vi "Create TopicFilter.vi"(5 "TopicFilter in":refnum<class "TopicFilter.lvclass">, 8 "error in (no error)":errorcluster, 11 "Topic Filter":string) -> (0 "error out":errorcluster, 3 "TopicFilter out":refnum<class "TopicFilter.lvclass">)   [LabVIEW 2013, in "MQTT Server.lvlib" / "TopicFilter.lvclass"]
uses:
  TopicFilter.lvclass
  TopicFilter.lvclass/TopicFilter.ctl
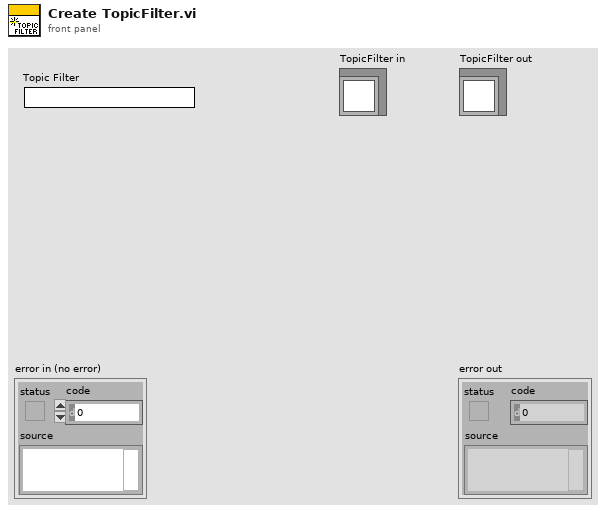
[diagram p1: front panel]
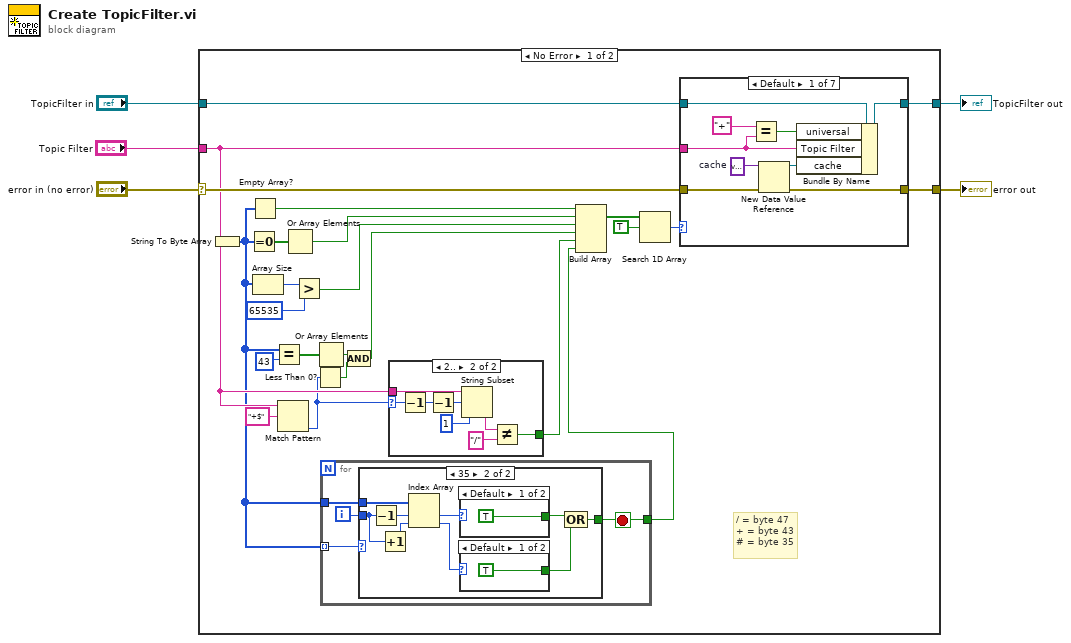
[diagram p0: block diagram]
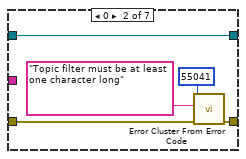
[diagram p6: hidden frame]
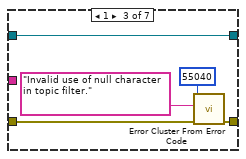
[diagram p7: hidden frame]
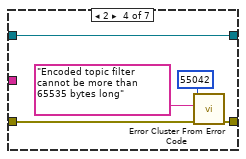
[diagram p8: hidden frame]
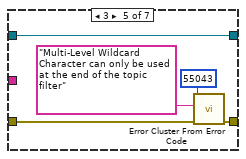
[diagram p9: hidden frame]
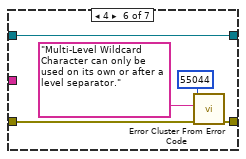
[diagram p10: hidden frame]
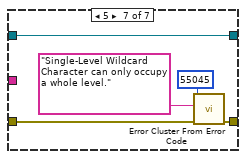
[diagram p11: hidden frame]
diagram:
  n1 = case shown="No Error" "error in (no error)" {
    selector: "error in (no error)" -> [w27 w93]
    tunnel: [w26 w93] -> w4
    tunnel: [w28 w92] -> w2
    tunnel: "TopicFilter in" -> [w29 w92]
    tunnel: "Topic Filter" -> [w10 _]
    frame No Error {
      # "/ = byte 47\n+ = byte 43\n# = byte 35"
      n2 = String To Byte Array(string=w10) -> (unsigned byte array=w7:u8[])
      n3 = Equal To 0?(x=w7) -> (x = 0?=w25:bool[])
      n4 = Empty Array?(array=w7) -> (empty?=w24:bool)
      n5 = Array Size(array=w7) -> (size(s)=w19:i32)
      n6 = Equal?(x=w7, y=u8 43) -> (x = y?=w14:bool[])
      n7 = Match Pattern(string=w10, regular expression="+$") -> (offset past match=w9:i32)  [unwired: 1 in, 3 out]
      n8 = Or Array Elements(Boolean array=w25) -> (logical OR=w23:bool)
      n9 = Greater?(x=w19, y=65535) -> (0:w17:bool)
      n10 = Less Than 0?(x=w9) -> (x < 0?=w12:bool)
      n11 = Or Array Elements(Boolean array=w14) -> (logical OR=w13:bool)
      n12 = for {
        tunnel: w7 -> [w33] mode=indexing
        tunnel: w7 -> [w32]
        tunnel: [w30] -> w6
        i -> [w31]
        stop <- w30 stop-if-true
        n13 = case shown="35" w33 {
          tunnel: w32 -> [_ w42]
          tunnel: w31 -> [_ w40]
          tunnel: [_ w34] -> w30
          frame Default {
          }
          frame 35 {
            n14 = Decrement(x=w40) -> (x-1=w41:i32)
            n15 = Increment(x=w40) -> (x+1=w39:i32)
            n16 = Index Array(array=w42, index #1=w41, index #2=w39) -> (element #1=w38:u8, element #2=w37:u8)
            n17 = case shown="Default" w38 {
              tunnel: [TRUE _] -> w36
              frame Default {
              }
              frame 0, 47 {
              }
            }
            n18 = case shown="Default" w37 {
              tunnel: [TRUE _] -> w35
              frame Default {
              }
              frame 0, 47 {
              }
            }
            n19 = Compound Arithmetic op=OR(w36, w35) -> (w34:bool)
          }
        }
      }
      n20 = Compound Arithmetic op=AND(w13, w12) -> (w11:bool)
      n21 = case shown="2.." w9 {
        selector: w9 -> [_ w48]
        tunnel: w10 -> [_ w52]
        tunnel: [_ w45] -> w8
        frame Default {
        }
        frame 2.. {
          n22 = Decrement(x=w48) -> (x-1=w51:i32)
          n23 = Decrement(x=w51) -> (x-1=w50:i32)
          n24 = String Subset(string=w52, offset (0)=w50, length (rest)=1 ("length (rest)")) -> (substring=w47:string)
          n25 = Not Equal?(x=w47, y="/" ("regular expression")) -> (x != y?=w45:bool)
        }
      }
      n26 = Build Array(w24, w23, w17, w11, w8, w6) -> (w21:bool[])
      n27 = Search 1D Array(1D array=w21, element=TRUE) -> (index of element=w20:i32)  [unwired: 1 in]
      n28 = case shown="Default" w20 {
        tunnel: w29 -> [w61 w66 w71 w76 w81 w86 w91]
        tunnel: [w60 w66 w71 w76 w81 w86 w91] -> w28
        tunnel: w27 -> [w57 w65 w70 w75 w80 w85 w90]
        tunnel: [w56 w64 w69 w74 w79 w84 w89] -> w26
        tunnel: w10 -> [w53 _ _ _ _ _ _]
        frame Default {
          w59 = variant  # cache
          n29 = Equal?(x="+" ("Topic Filter"), y=w53) -> (x = y?=w54:bool)
          n30 = New Data Value Reference(data value=w59, error in=w57) -> (data value reference=w58:refnum<data-value>, error out=w56:errorcluster)
          n31 = Bundle By Name(cluster=w61, "universal"=w54, "Topic Filter"=w53, "cache"=w58) -> (w60:refnum<class "TopicFilter.lvclass">)
        }
        frame 0 {
          n32 = call <vilib>:"Error Cluster From Error Code.vi"("error in (no error)"=w65, "error message (\"\")"="Topic filter must be at least one character long" ("error message (\"\")"), "error code (0)"=55041) -> ("error out"=w64:errorcluster)  [unwired: 6 in]
        }
        frame 1 {
          n33 = call <vilib>:"Error Cluster From Error Code.vi"("error in (no error)"=w70, "error message (\"\")"="Invalid use of null character in topic filter." ("error message (\"\")"), "error code (0)"=55040) -> ("error out"=w69:errorcluster)  [unwired: 6 in]
        }
        frame 2 {
          n34 = call <vilib>:"Error Cluster From Error Code.vi"("error in (no error)"=w75, "error message (\"\")"="Encoded topic filter cannot be more than 65535 bytes long" ("error message (\"\")"), "error code (0)"=55042) -> ("error out"=w74:errorcluster)  [unwired: 6 in]
        }
        frame 3 {
          n35 = call <vilib>:"Error Cluster From Error Code.vi"("error in (no error)"=w80, "error message (\"\")"="Multi-Level Wildcard Character can only be used at the end of the topic filter" ("error message (\"\")"), "error code (0)"=55043) -> ("error out"=w79:errorcluster)  [unwired: 6 in]
        }
        frame 4 {
          n36 = call <vilib>:"Error Cluster From Error Code.vi"("error in (no error)"=w85, "error message (\"\")"="Multi-Level Wildcard Character can only be used on its own or after a level separator." ("error message (\"\")"), "error code (0)"=55044) -> ("error out"=w84:errorcluster)  [unwired: 6 in]
        }
        frame 5 {
          n37 = call <vilib>:"Error Cluster From Error Code.vi"("error in (no error)"=w90, "error message (\"\")"="Single-Level Wildcard Character can only occupy a whole level." ("error message (\"\")"), "error code (0)"=55045) -> ("error out"=w89:errorcluster)  [unwired: 6 in]
        }
      }
    }
    frame Error {
    }
  }
  "error out" <- w4
  "TopicFilter out" <- w2
